vi "auto time.vi"() -> ()   [LabVIEW 2016]
panel:
  out "4U70 71M4":dbl
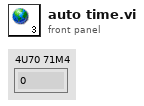
[diagram p1: front panel]
diagram:
